vi "Launcher.vi"   [LabVIEW 2019]
uses:
  <vilib>/ActorFramework/Actor/Actor.lvclass
  EmulatorActor/EmulatorActor/EmulatorActor.lvclass
  DigitiserActor/DigitiserActor/DigitiserActor.lvclass
  C:/Program Files (x86)/National Instruments/LabVIEW 2019/vi.lib/ActorFramework/Actor/Actor.lvclass
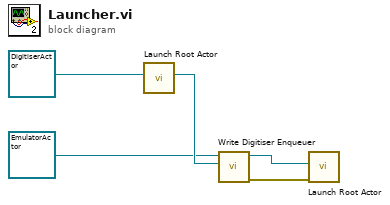
[diagram p0: block diagram]
diagram:
  n1 = call <vilib>:"Launch Root Actor.vi"("Actor"=refnum<class "DigitiserActor.lvclass"> refnum ("DigitiserActor.lvlib:DigitiserActor.lvclass")) -> ("Actor's Enqueuer"=w3:refnum<class "Message Enqueuer.lvclass">)  [unwired: 9 in, 1 out]
  n2 = call "Write Digitiser Enqueuer.vi"("Actor Framework:Message Enqueuer"=w3, "EmulatorActor in"=refnum<class "EmulatorActor.lvclass"> refnum ("EmulatorActor.lvlib:EmulatorActor.lvclass")) -> ("error out"=w4:errorcluster, "EmulatorActor out"=w5:refnum<class "EmulatorActor.lvclass">)  [unwired: 8 in]
  n3 = call <vilib>:"Launch Root Actor.vi"("error in (no error)"=w4, "Actor"=w5) -> ()  [unwired: 8 in, 2 out]
